vi "Prompt User.vi"(8 "error in":errorcluster, 11 "Message":string) -> (0 "error out":errorcluster, 2 "choice":bool)   [LabVIEW 2015]
doc: "This VI is the prompt that will show to the user on an error. The color for the top box and the borders for the two buttons is loaded from the config file. If the config file is not present, then the Windows Metro Blue RGB color is used by default. \n\nInputs:\n-Message [string] - the error message\n-error in\n\nOutputs:\n-choice [Boolean] - the user's choice to continue or exit the program\n-error out\n________________________________________________________________________________\n<b>Code Developed By:</b>\nDaniel Coons\nTechnology Service Corporation\n1983 S Liberty Drive\nBloomington, IN 47403\nPhone: 812 558-7100\ndaniel.coons@tsc.com\nwww.tsc.com\n\n<b>Date Created:</b> 11 AUG 2014\n<b>Date Updated:</b> 20 AUG 2014"
uses:
  <vilib>/Utility/config.llb/Read Key (String).vi
  <vilib>/Utility/config.llb/NI_LVConfig.lvlib
panel:
  in  "X":bool
  in  "exit":bool
  in  "continue":bool
  # "An error has occurred:"
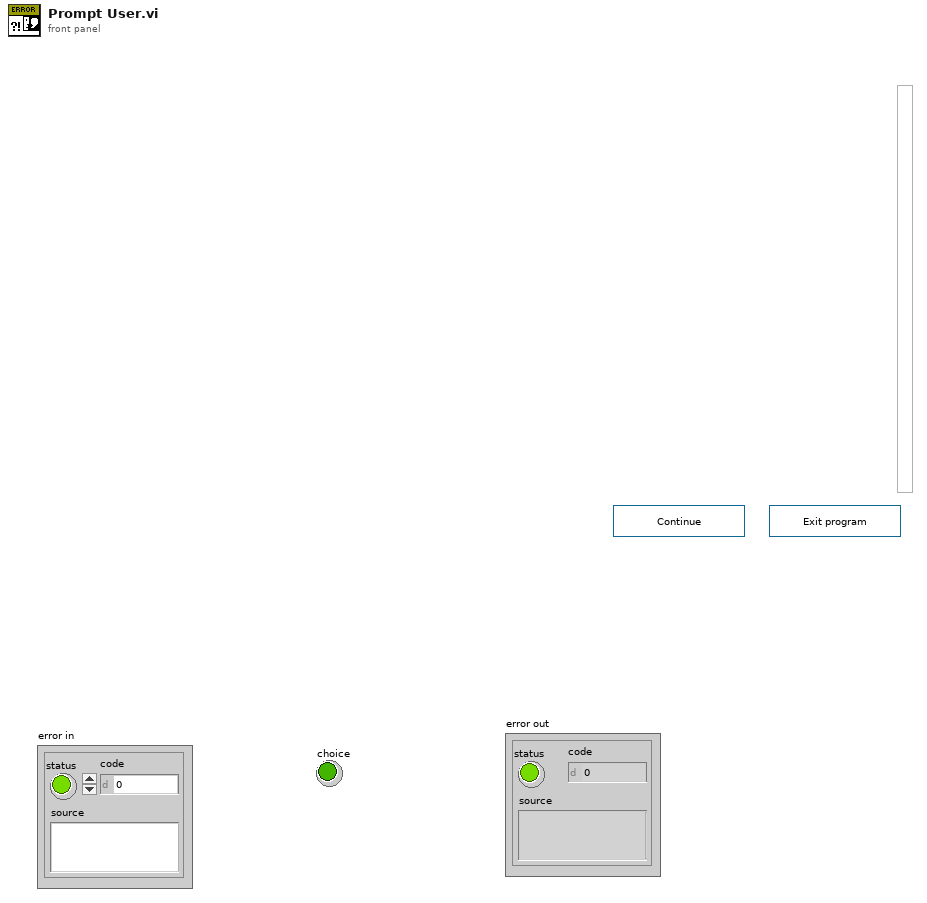
[diagram p1: front panel]
types:
  T1 = typedef "NI_LVConfig.lvlib/Config Data RefNum.ctl" = refnum<k1>
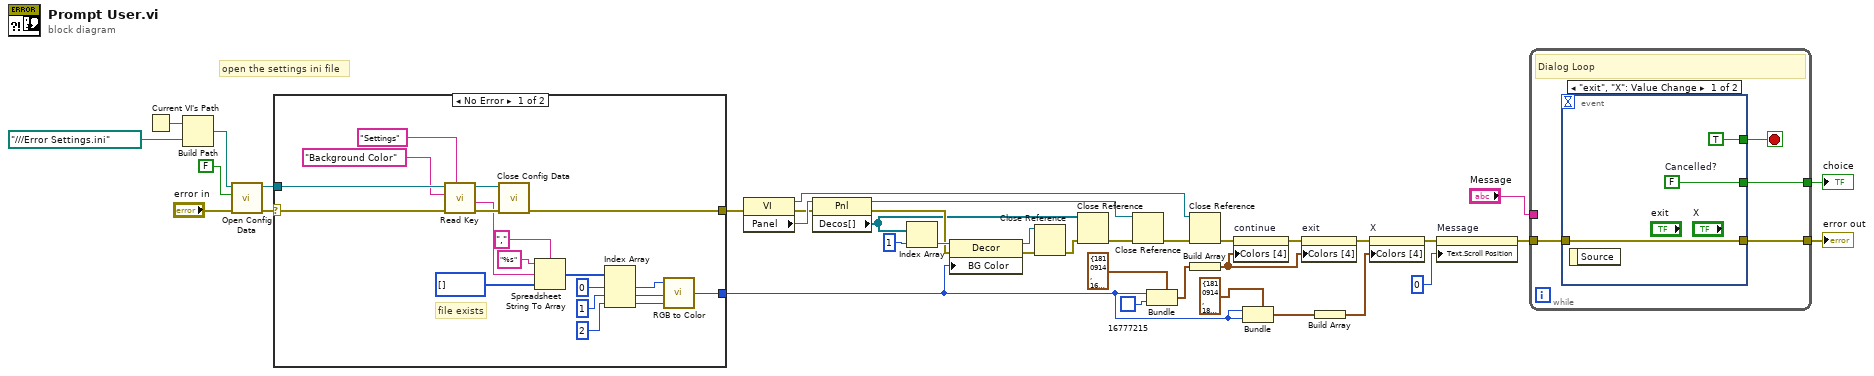
[diagram p0: block diagram]
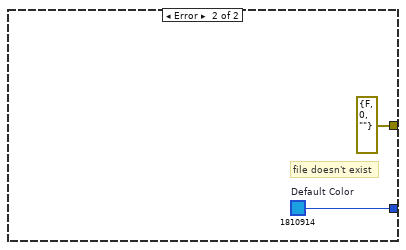
[diagram p2: hidden frame]
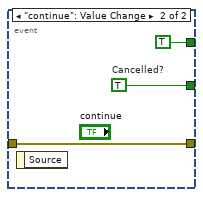
[diagram p3: hidden frame]
diagram:
  # "open the settings ini file"
  n1 = Current VI's Path() -> (path=w15:path)
  n2 = Build Path(base path=w15, name or relative path=path "../../../Error Settings.ini") -> (appended path=w14:path)
  n3 = call <vilib>:"Open Config Data.vi"("error in (no error)"="error in", "create file if necessary (T)"=FALSE, "configuration file path"=w14) -> ("error out"=w1:errorcluster, "refnum"=w13:T1)  [unwired: 6 in, 1 out]
  n4 = case shown="No Error" w1 {
    selector: w1 -> [w39 _]
    tunnel: w13 -> [w57 _]
    tunnel: [w41 w59] -> w3
    tunnel: [w40 errorcluster {"status"=FALSE, "code"=0, "source"=""} ("error out")] -> w2
    frame No Error {
      # "file exists"
      n5 = call-poly <vilib>:"Read Key.vi"("section"="Settings", "error in (no error)"=w39, "key"="Background Color", "refnum"=w57) -> ("error out"=w54:errorcluster, "value"=w50:string, "refnum out"=w53:T1)  [unwired: 4 in, 1 out]
      n6 = call <vilib>:"Close Config Data.vi"("error in (no error)"=w54, "refnum"=w53) -> ("error out"=w40:errorcluster)  [unwired: 8 in, 1 out]
      n7 = Spreadsheet String To Array(delimiter (Tab)=",", format string="%s", spreadsheet string=w50, array type (2D Dbl)=u8[] []) -> (array=w48:u8[])
      n8 = Index Array(array=w48, index #1=0 ("index"), index #2=1 ("index"), index #3=2 ("index")) -> (element #1=w42:u8, element #2=w44:u8, element #3=w43:u8)
      n9 = call <vilib>:"RGB to Color.vi"("B"=w43, "G"=w44, "R"=w42) -> ("Color"=w41:u32)
    }
    frame Error {
      w59 = u32 1810914  # Default Color
      # "file doesn't exist"
    }
  }
  n10 = property class="VI"(error in=w2) -> (reference out=w20:refnum<vi>, error out=w26:errorcluster, "Panel"=w33:refnum<vi>)  [unwired: 1 in]
  n11 = property class="Pnl"(reference=w33, error in=w26) -> (reference out=w22:refnum<vi>, error out=w27:errorcluster, "Decos[]"=w23:refnum<vi>[])
  n12 = Index Array(array=w23, index=1) -> (element=w32:refnum<vi>)
  n13 = property class="Decor"(reference=w32, error in=w27, "BG Color"=w3) -> (reference out=w28:refnum<vi>, error out=w29:errorcluster)
  n14 = Close Reference(reference=w28, error in (no error)=w29) -> (error out=w25:errorcluster)
  n15 = Close Reference(reference=w23, error in (no error)=w25) -> (error out=w24:errorcluster)
  n16 = Close Reference(reference=w22, error in (no error)=w24) -> (error out=w21:errorcluster)
  n17 = Bundle(cluster=cluster{u32, u32} {1810914, 16777215}, w3, u32 16777215) -> (w8:cluster{u32, u32})
  n18 = Close Reference(reference=w20, error in (no error)=w21) -> (error out=w17:errorcluster)
  n19 = Build Array(w8) -> (w7:cluster{u32, u32}[])
  n20 = property on="continue" class="Bool (strict)"(error in=w17, "Colors [4]"=w7) -> (error out=w18:errorcluster)  [unwired: 1 in, 1 out]
  n21 = Bundle(cluster=cluster{u32, u32} {1810914, 1810914}, w3, w3) -> (w5:cluster{u32, u32})
  n22 = property on="exit" class="Bool (strict)"(error in=w18, "Colors [4]"=w7) -> (error out=w19:errorcluster)  [unwired: 1 in, 1 out]
  n23 = Build Array(w5) -> (w4:cluster{u32, u32}[])
  n24 = property on="X" class="Bool (strict)"(error in=w19, "Colors [4]"=w4) -> (error out=w30:errorcluster)  [unwired: 1 in, 1 out]
  n25 = property on="Message" class="Str"(error in=w30, "Text.Scroll Position"=u32 0) -> (error out=w34:errorcluster)  [unwired: 1 in, 1 out]
  n26 = while {
    tunnel: [w62] -> w38
    tunnel: "Message" -> [_]
    tunnel: [w61] -> w36
    tunnel: w34 -> [w60]
    stop <- w63 stop-if-true
    # "Dialog Loop"
    n27 = event shown="[0] \"exit\", \"X\": Value Change" {
      selector: _ -> [_ _]
      dyn-events: _ -> [_ _]
      timeout: _ -> [_ _]
      tunnel: [TRUE ("Stop?") TRUE ("Stop?")] -> w63
      tunnel: [w66 w69] -> w62
      tunnel: [w64 w67] -> w61
      tunnel: w60 -> [w64 w67]
      event "exit", "X": Value Change {
        w66 = FALSE  # Cancelled?
        n28 = event-data() -> ()  [unwired: 1 in, 1 out]
      }
      event "continue": Value Change {
        w69 = TRUE  # Cancelled?
        n29 = event-data() -> ()  [unwired: 1 in, 1 out]
      }
    }
  }
  "choice" <- w38
  "error out" <- w36
